vi "addRecursive.vi"(1 "Command URL in":string, 2 "Parameter Key":string[](array[string]), 3 "Parameter Value":string[](array[string]), 4 "Finish? in":bool) -> (15 "Command URL out":string, 16 "Parameter Key Out":string[](array[string]), 17 "Parameter Value Out":string[](array[string]), 18 "Finish? out":bool)   [LabVIEW 2019, in "PF_API.lvclass"]
uses:
  PF_API.lvclass
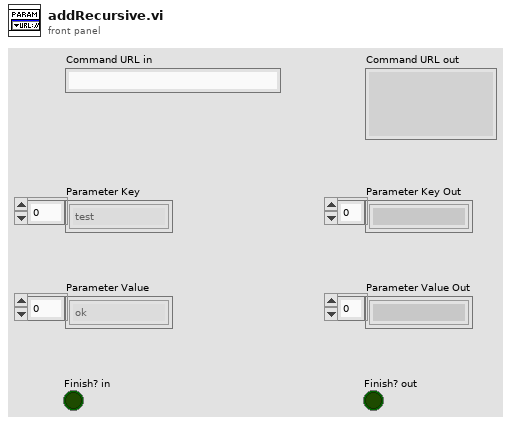
[diagram p1: front panel]
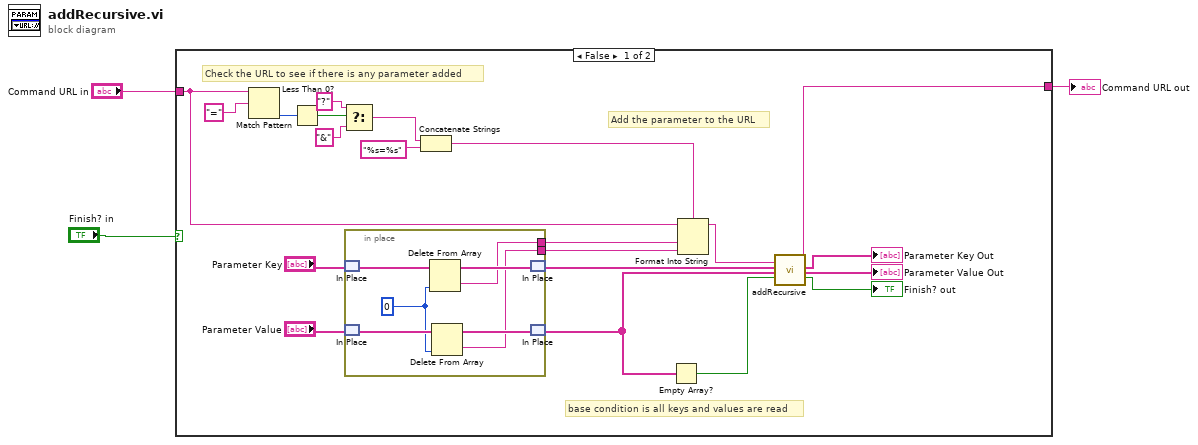
[diagram p0: block diagram]
diagram:
  n1 = case shown="False" "Finish? in" {
    tunnel: [w10 w32] -> w3
    tunnel: "Command URL in" -> [w12 w32]
    frame False {
      # "base condition is all keys and values are read"
      # "Check the URL to see if there is any parameter added"
      # "Add the parameter to the URL"
      n2 = Match Pattern(string=w12, regular expression="=") -> (offset past match=w21:i32)  [unwired: 1 in, 3 out]
      n3 = Less Than 0?(x=w21) -> (x < 0?=w20:bool)
      n4 = Select(t="?" ("regular expression"), s=w20, f="&" ("regular expression")) -> (s? t:f=w17:string)
      n5 = in-place {
        in-place-border: [w27] -> w14
        in-place-border: [w26] -> w13
        w25 = 0 ("index")
        n6 = in-place-match #1("Parameter Key") -> (w31:string[])
        n7 = in-place-match #2("Parameter Value") -> (w29:string[])
        n8 = Delete From Array(array=w31, index=w25) -> (deleted portion=w27:string, array with subset deleted=w30:string[])  [unwired: 1 in]
        n9 = Delete From Array(array=w29, index=w25) -> (deleted portion=w26:string, array with subset deleted=w28:string[])  [unwired: 1 in]
        n10 = in-place-match #1(w30) -> (w9:string[])
        n11 = in-place-match #2(w28) -> (w8:string[])
      }
      n12 = Concatenate Strings(w17, "%s=%s" ("format string")) -> (w23:string)
      n13 = Empty Array?(array=w8) -> (empty?=w7:bool)
      n14 = Format Into String(format string=w23, initial string=w12, w14, w13) -> (resulting string=w11:string)  [unwired: 1 in, 1 out]
      n15 = call "addRecursive.vi"("Command URL in"=w11, "Parameter Key"=w9, "Parameter Value"=w8, "Finish? in"=w7) -> ("Command URL out"=w10:string, "Parameter Key Out"=→"Parameter Key Out":string[], "Parameter Value Out"=→"Parameter Value Out":string[], "Finish? out"=→"Finish? out":bool)  [unwired: 12 in]
    }
    frame True {
    }
  }
  "Command URL out" <- w3
